vi "NIReadGlobal.vi"() -> ()   [LabVIEW 2019]
panel:
  in  "NI Read Values":T1
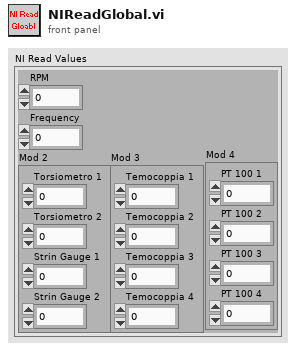
[diagram p1: front panel]
types:
  T1 = cluster{"RPM":dbl, "Frequency":dbl, "Mod 2":cluster{"Torsiometro 1":dbl, "Torsiometro 2":dbl, "Strin Gauge 1":dbl, "Strin Gauge 2":dbl}, "Mod 3":cluster{"Temocoppia 1":dbl, "Temocoppia 2":dbl, "Temocoppia 3":dbl, "Temocoppia 4":dbl}, "Mod 4":cluster{"PT 100 1":dbl, "PT 100 2":dbl, "PT 100 3":dbl, "PT 100 4":dbl}}
diagram:
